vi "SetShuntType.vi"(6 "time out":u32, 9 "Shunt Type":u8(ring) items=["100A"=1, "200A"=2, "300A"=3, "400A"=4, "500A"=5, "600A"=6, "50A"=11], 10 "类型":u32(ring)=4 items=["PCI5121"=1, "PCI9810"=2, "USBCAN1"=3, "USBCAN2"=4, "PCI9820"=5, "CAN232"=6, "PCI5110"=7, "CANLite(mini)"=8, "ISA9620"=9, "ISA5420"=10, "PC104CAN"=11, "CANET"=17, "DNP9810"=13, "USBCAN-E-U"=20, "USBCAN-2E-U"=21], 12 "设备索引":u32(ring) items=["0", "1", "2", "3", "4", "5", "6", "7", "8", "9", "10", "11", "12", "13", "14", "15", ""], 16 "CAN路数":u32(ring) items=["0", "1"]) -> (20 "set ok?":bool)   [LabVIEW 2013]
uses:
  AutoBurn/Settings/ControlCAN.dll
panel:
  out "VCI_CAN_OBJ_T":T1 {"ID" format="%x"}
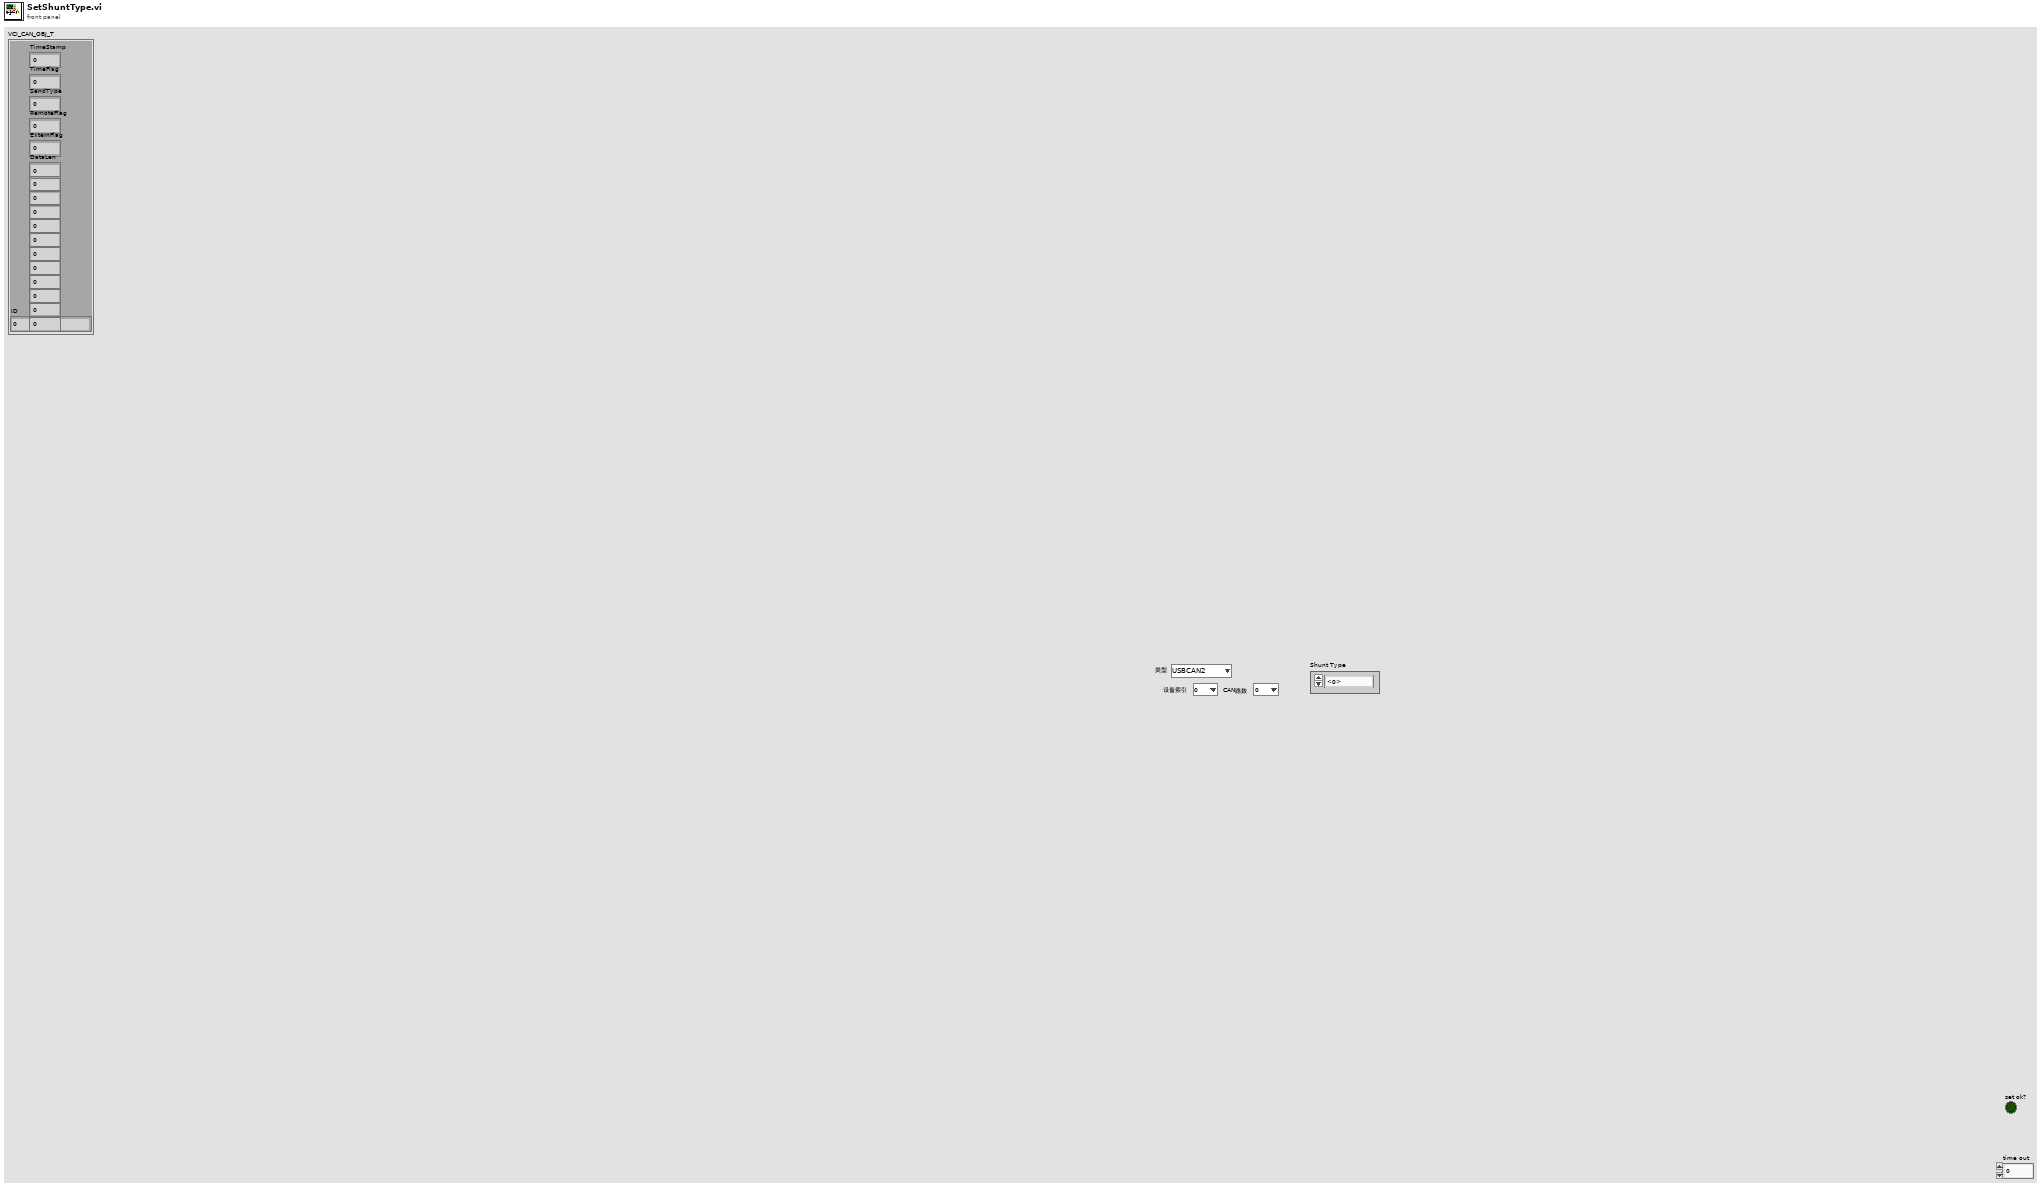
[diagram p1: front panel]
types:
  T1 = cluster{"ID":u32, "TimeStamp":u32, "TimeFlag":u8, "SendType":u8, "RemoteFlag":u8, "ExternFlag":u8, "DataLen":u8, u8, u8, u8, u8, u8, u8, u8, u8, u8, u8, u8}
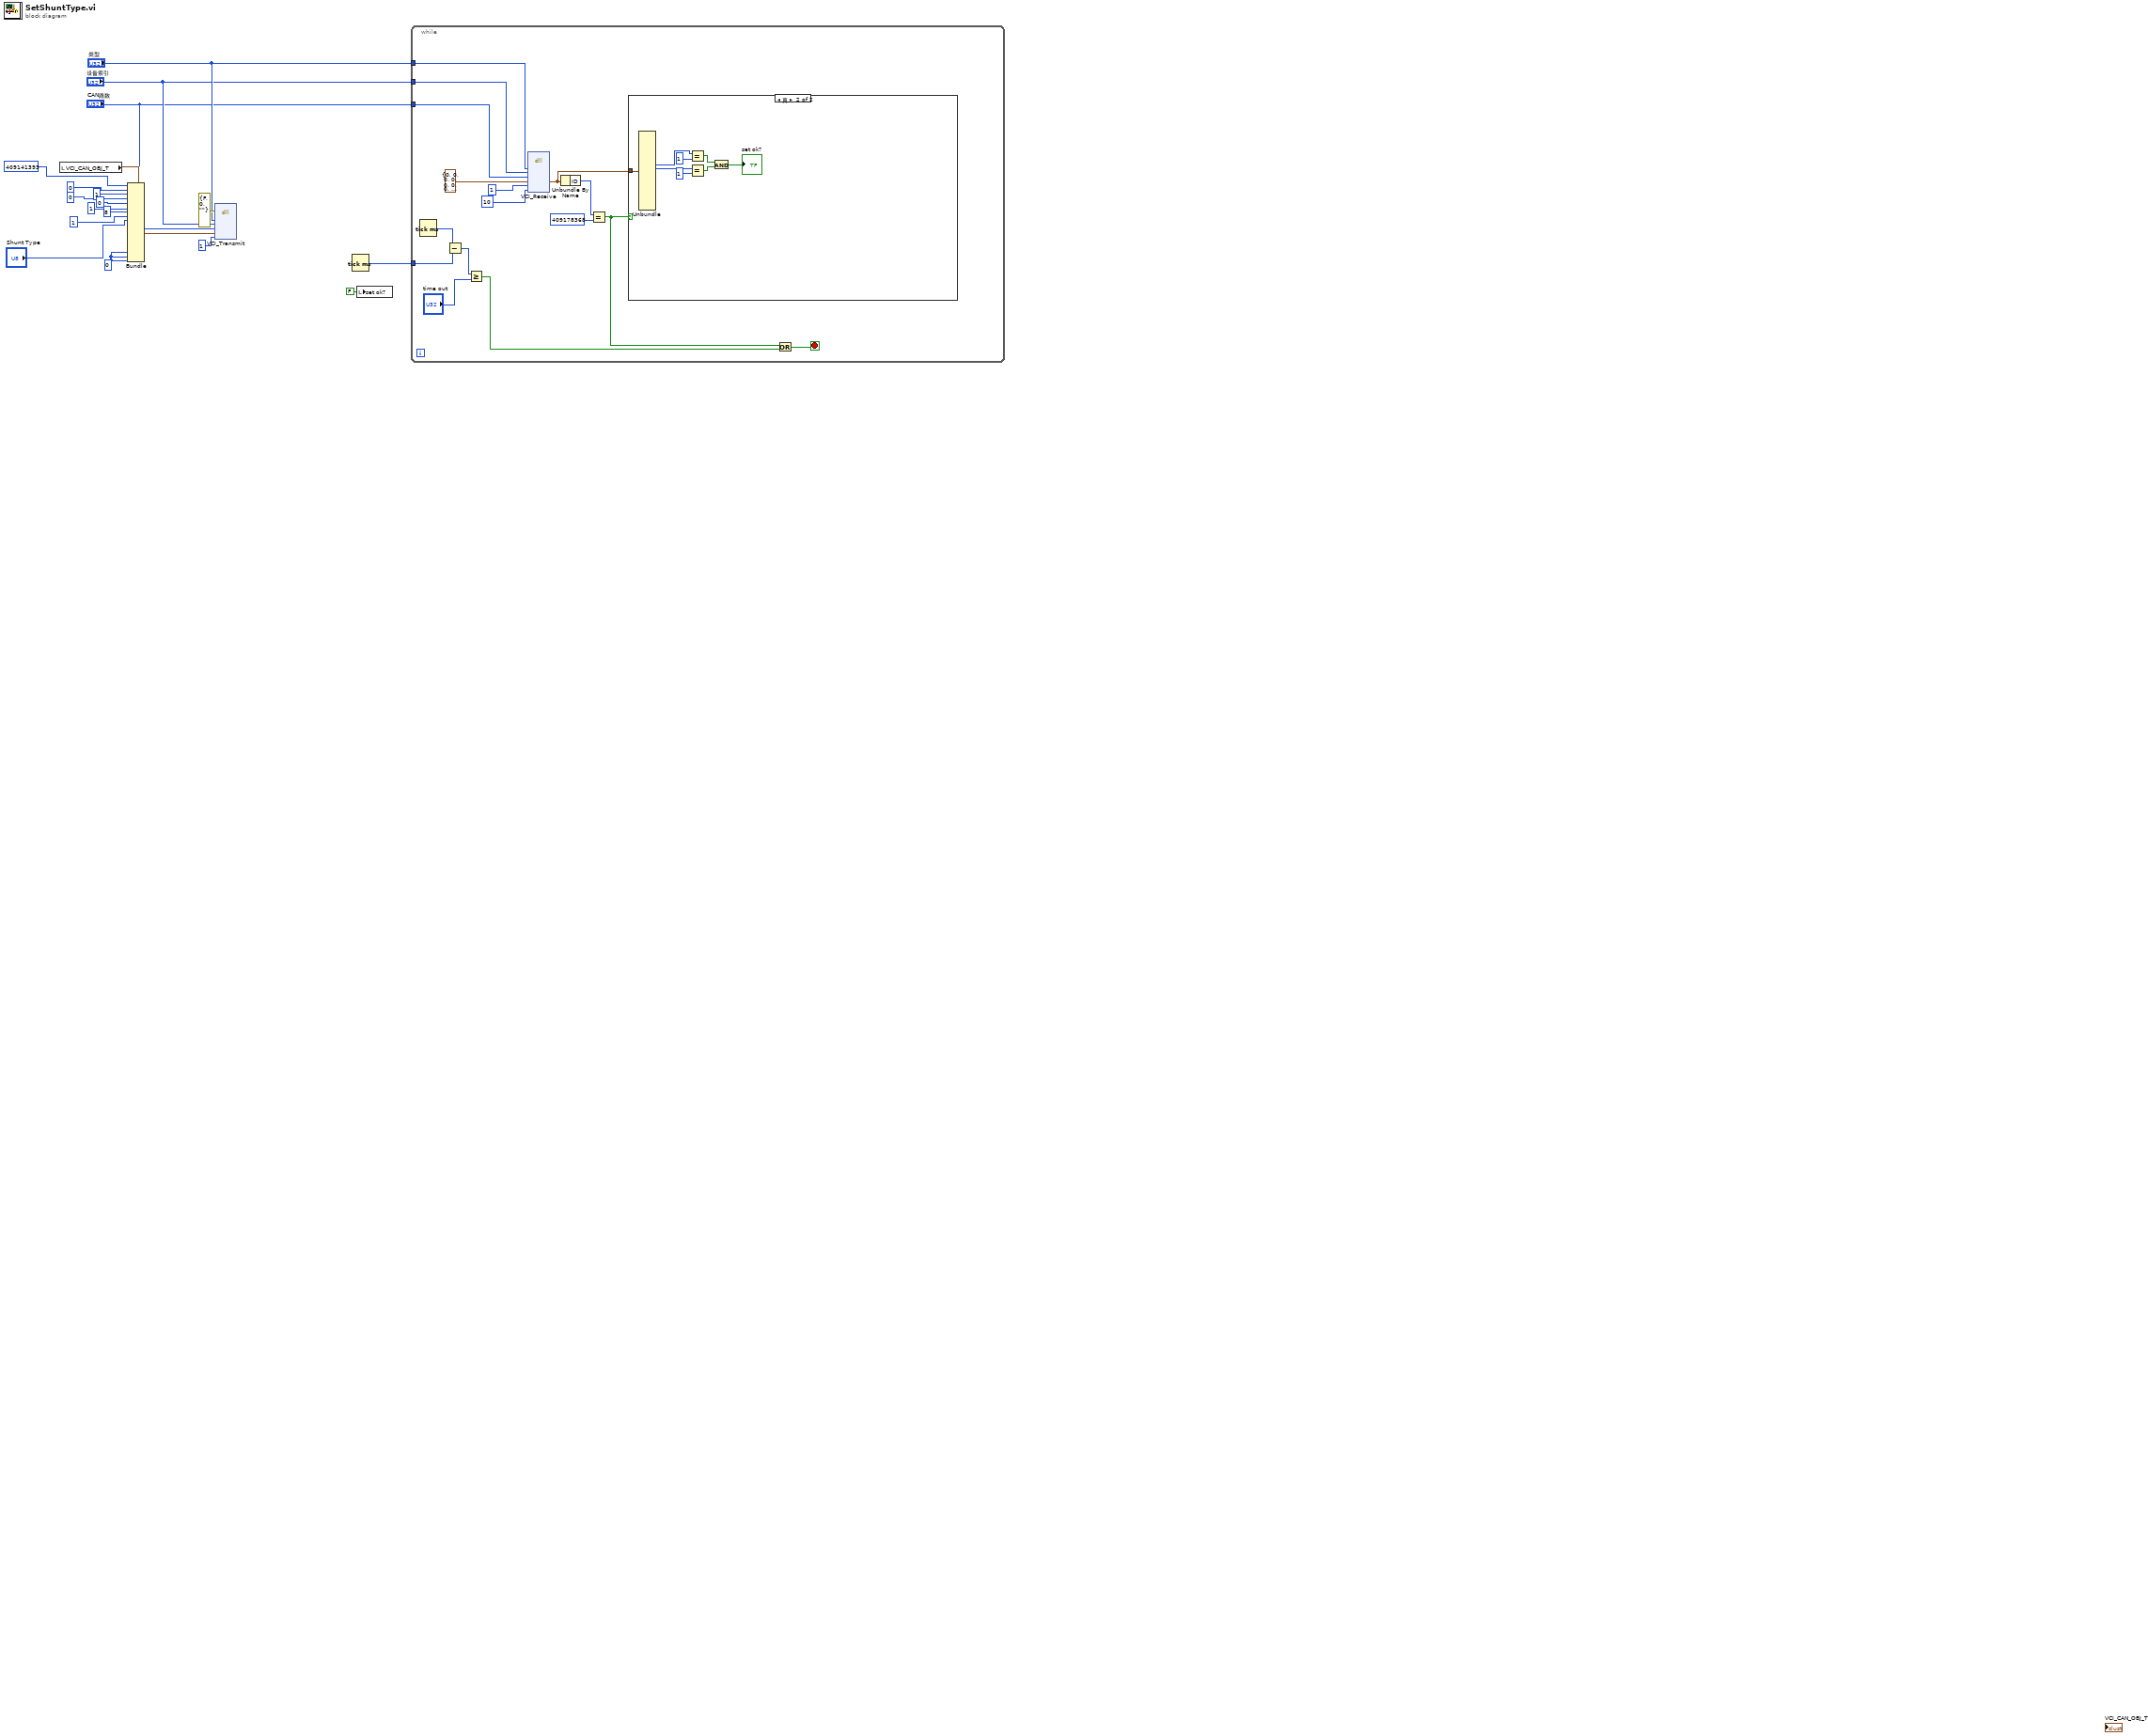
[diagram p0: block diagram]
diagram:
  w11 = u8 0 ("元素")
  n1 = local read "VCI_CAN_OBJ_T"() -> (w15:T1)
  n2 = Bundle(cluster=w15, "ID"=u32 409141393 ("RemoteFlag"), "TimeStamp"=u8 0 ("RemoteFlag"), "TimeFlag"=u8 1, "SendType"=u8 0 ("DataLen"), "RemoteFlag"=u8 0, "ExternFlag"=u8 1, "DataLen"=u8 8, u8 1, "Shunt Type", w11, w11, w11) -> (w16:T1)  [unwired: 6 in]
  n3 = dll-call lib="F:/Bluewave New Energy/SVN_Work/AutoTest_TestStand/trunk/AutoTest_TestStand/Driver/ZlgCan/BHN01/AutoBurn/Settings/ControlCAN.dll" fn="VCI_Transmit"(error in=errorcluster {"status"=FALSE, "code"=0, "source"=""} ("错误输入（无错误）"), "DeviceType"="类型", "DeviceInd"="设备索引", "CANInd"="CAN路数", "pSend"=w16, "Len"=u32 1) -> ()  [unwired: 4 in, 6 out]
  n4 = Tick Count (ms)() -> (millisecond timer value=w19:u32)
  n5 = local write "set ok?"(FALSE ("x = y?")) -> ()
  n6 = while {
    tunnel: w19 -> [w31]
    tunnel: "类型" -> [w22]
    tunnel: "设备索引" -> [w21]
    tunnel: "CAN路数" -> [w20]
    stop <- w25 stop-if-true
    n7 = Tick Count (ms)() -> (millisecond timer value=w32:u32)
    n8 = Subtract(x=w32, y=w31) -> (x-y=w30:u32)
    n9 = Greater Or Equal?(x=w30, y="time out") -> (x >= y?=w26:bool)
    n10 = dll-call lib="F:/Bluewave New Energy/SVN_Work/AutoTest_TestStand/trunk/AutoTest_TestStand/Driver/ZlgCan/BHN01/AutoBurn/Settings/ControlCAN.dll" fn="VCI_Receive"("DeviceType"=w22, "DeviceInd"=w21, "CANInd"=w20, "pReceive"=T1 {"ID"=0, "TimeStamp"=0, "TimeFlag"=0, "SendType"=0, "RemoteFlag"=0, "ExternFlag"=0, "DataLen"=0, 0, 0, 0, 0, 0, 0, 0, 0, 0, 0, 0}, "Len"=u32 1, "WaitTime"=10) -> ("pReceive"=w24:T1)  [unwired: 8 in, 3 out]
    n11 = Unbundle By Name(w24) -> ("ID"=w28:u32)
    n12 = Equal?(x=w28, y=u32 409178368) -> (x = y?=w27:bool)
    n13 = case shown="真" w27 {
      tunnel: w24 -> [_ w43]
      frame False {
      }
      frame True {
        n14 = Unbundle(w43) -> (w39:u8, w42:u8)  [unwired: 16 out]
        n15 = Equal?(x=w39, y=u8 1) -> (x = y?=w37:bool)
        n16 = Equal?(x=w42, y=u8 1) -> (x = y?=w38:bool)
        n17 = And(x=w37, y=w38) -> (x .and. y?=→"set ok?":bool)
      }
    }
    n18 = Or(x=w27, y=w26) -> (x .or. y?=w25:bool)
  }
